vi "习题4.4.vi"() -> ()   [LabVIEW 2018]
panel:
  in  "温度 2":dbl(slide) scale=-50.0..50.0
  in  "温度":dbl(slide) scale=-50.0..50.0
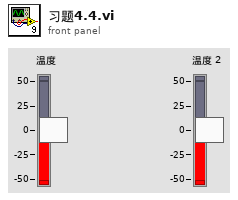
[diagram p1: front panel]
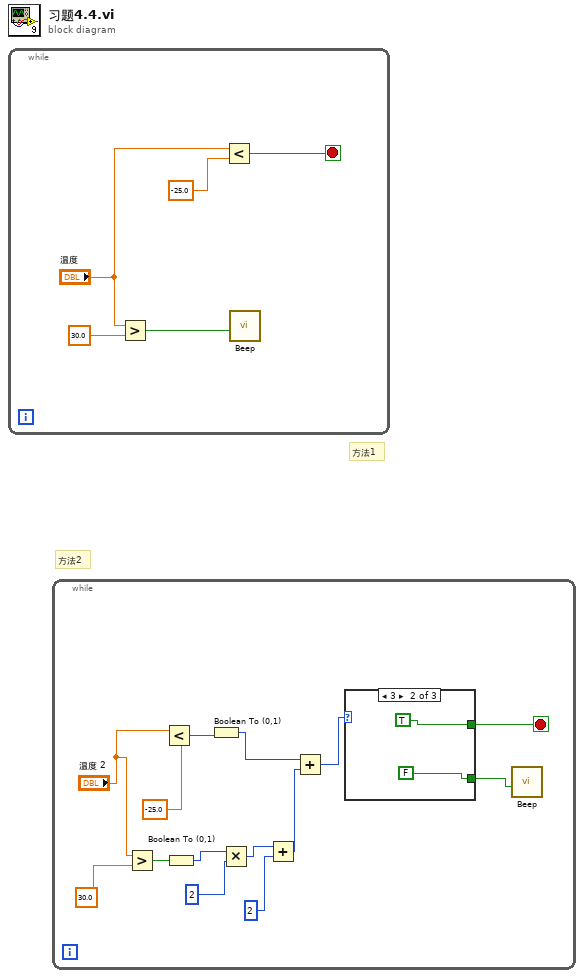
[diagram p0: block diagram]
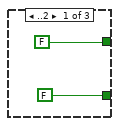
[diagram p2: hidden frame]
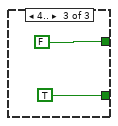
[diagram p3: hidden frame]
diagram:
  # "方法1"
  # "方法2"
  n1 = while {
    stop <- w2 stop-if-true
    n2 = Greater?(x="温度", y=30.0) -> (0:w1:bool)
    n3 = Less?(x="温度", y=-25.0) -> (x < y?=w2:bool)
    n4 = call <vilib>:"Beep.vi"("use system alert? (T)"=w1) -> ()  [unwired: 11 in]
  }
  n5 = while {
    stop <- w6 stop-if-true
    n6 = Greater?(x="温度 2", y=30.0) -> (0:w16:bool)
    n7 = Less?(x="温度 2", y=-25.0) -> (x < y?=w12:bool)
    n8 = Boolean To (0,1)(Boolean=w16) -> (0, 1=w15:i16)
    n9 = Boolean To (0,1)(Boolean=w12) -> (0, 1=w11:i16)
    n10 = Multiply(x=w15, y=i16 2) -> (x*y=w10:i16)
    n11 = Add(x=w10, y=i16 2) -> (x+y=w9:i16)
    n12 = Add(x=w11, y=w9) -> (x+y=w7:i16)
    n13 = case shown="3" w7 {
      tunnel: [FALSE TRUE FALSE] -> w6
      tunnel: [FALSE FALSE TRUE] -> w8
      frame ..2 {
      }
      frame 3 {
      }
      frame 4.. {
      }
    }
    n14 = call <vilib>:"Beep.vi"("use system alert? (T)"=w8) -> ()  [unwired: 11 in]
  }
